vi "SubVI TX Transmitter Init.vi"(8 "错误输入":errorcluster, 10 "IQ数据":cluster{"t0":dbl, "dt":dbl, "Y":cdb[]}) -> (0 "错误输出":errorcluster, 2 "缩放和填充IQ数据":cluster{"t0":dbl, "dt":dbl, "Y":cdb[]})   [LabVIEW 2015]
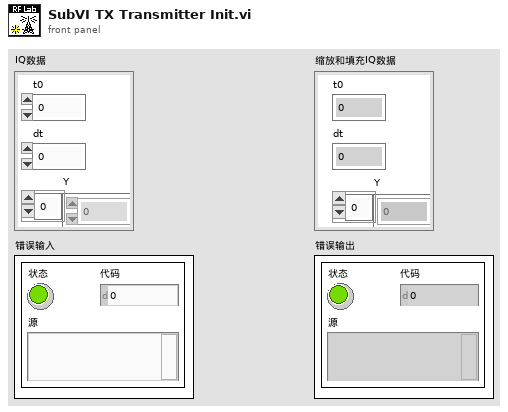
[diagram p1: front panel]
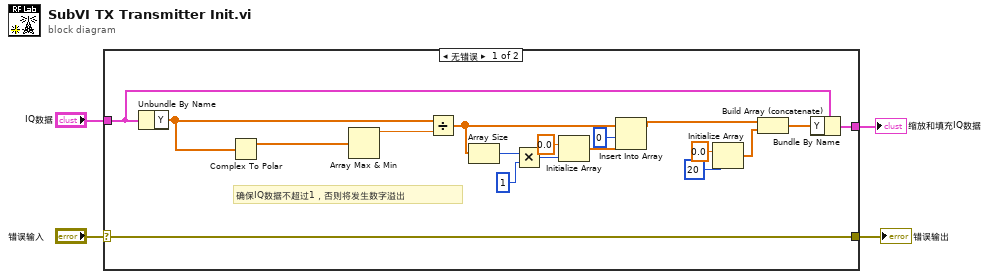
[diagram p0: block diagram]
diagram:
  n1 = case shown="无错误" "错误输入" {
    selector: "错误输入" -> [w5 w23]
    tunnel: "IQ数据" -> [w22 _]
    tunnel: [w21 _] -> w3
    tunnel: [w5 w23] -> w1
    frame No Error {
      # "确保IQ数据不超过1，否则将发生数字溢出"
      n2 = Unbundle By Name(w22) -> ("Y"=w20:cdb[])
      n3 = Complex To Polar(r * e^(i*theta)=w20) -> (r=w19:dbl[])  [unwired: 1 out]
      n4 = Array Max & Min(array=w19) -> (max value=w18:dbl)  [unwired: 3 out]
      n5 = Divide(x=w20, y=w18) -> (x/y=w11:cdb[])
      n6 = Array Size(array=w11) -> (size(s)=w14:i32)
      n7 = Multiply(x=w14, y=1) -> (x*y=w13:i32)
      n8 = Initialize Array(0.0 ("element"), w13) -> (w15:dbl[])
      n9 = Insert Into Array(array=w11, index=0, new element=w15) -> (w8:cdb[])
      n10 = Initialize Array(0.0 ("element"), 20 ("dimension size")) -> (w9:dbl[])
      n11 = Build Array (concatenate)(w8, w9) -> (w7:cdb[])
      n12 = Bundle By Name(cluster=w22, "Y"=w7) -> (w21:cluster{"t0":dbl, "dt":dbl, "Y":cdb[]})
    }
    frame Error {
    }
  }
  "缩放和填充IQ数据" <- w3
  "错误输出" <- w1
